vi "LDA_cold_wire_Corr_with_ Displacement.vi"() -> (5 "Plug in titles":string[](array[string]), 7 "Plug in values":string[](array[string]))   [LabVIEW 2021]
uses:
  Controls/Inst_type.ctl
  Globals/Meas_global.vi
  <vilib>/Analysis/NI_AALBase.lvlib
panel:
  out "Cold Wire/FFID Index":i32[](array[numeric])
  out "Maximum Delay Time (s)":dbl=0.02 format="%.3f"
  out "X Displacement (mm) Used":dbl
  in  "Default X Displacement (mm)":dbl=4.0
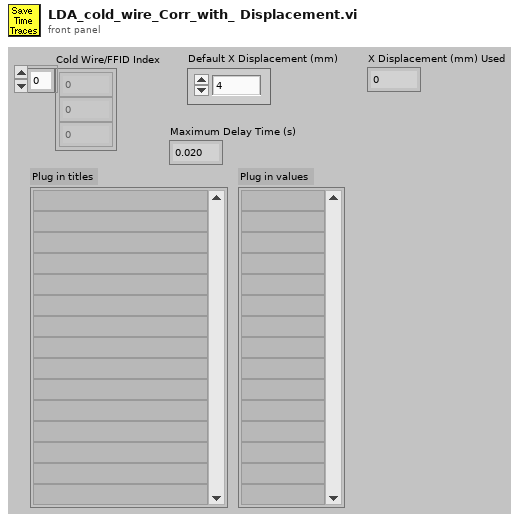
[diagram p1: front panel]
types:
  T1 = typedef "Analysis_info_cluster.ctl" = cluster{"Colour":u32, "Inst type":T2, "Inst name":string, "Symbol":string, "Code name":string, "Extra Info":string, "Inst Array":T3, "Extra Titles":string[], "Extra Values":string[], "U":dbl, "u^2":dbl, "u^3":dbl, "u^4":dbl, "Skew_u":dbl, "Kurt_u":dbl, "Sd Error in Mean":dbl, "% u'/U":dbl, "X":dbl, "Y":dbl, "Z":dbl, "Timescale integral Estimate":dbl, "Sd Error in Variance":dbl, "Calib File":path, "Calib Constants":dbl[], "Output Position":bool, "Stats":enum16{"None", "Basic", "Full"}, "Av Sampling Rate":dbl, "Av No of Samples":dbl, "Total Meas Time (s)":dbl, "ADAM Ch Name":string, "Max value":dbl, "Min value":dbl, "Req Sample Rate Hz":dbl, "Sync Delay Time (s)":dbl, "Ch No":i16, "Device":string, "Use Latest Calib":bool, "Port":string, "Metadata Ch Names":string[], "Metadata Ch Values":string[], "Label":string}
  T2 = typedef "Inst_type.ctl" = enum16{"Raw voltage", "Raw with zero offsetting", "Propeller anemometer", "Pressure Transducer", "Pitot-static tube", "Hot wire", "Cross wire 1", "Cross wire 2", "Generic Linear", "Generic Polynomial", "Generic BackPoly", "Fast FID", "Thermocouple", "Cold wire", "Pulsed Wire", "LDA Vel", "LDA Tran time", "LDA Arr time", "Microphone"}
  T3 = typedef "Instrument_Array.ctl" = enum16{"PWA", "LDA", "Analogue"}
  T4 = typedef "Time_Trace_Cluster.ctl" = cluster{"Weighting":dbl[], "Voltage":dbl[], "Eng Values":dbl[]}
  T5 = typedef "Cross_Moments_Shift_Cluster.ctl" = cluster{"Stats":dbl[], "Resampled No of Samples":i32, "Resampled delta T":dbl, "Cross Correlation":dbl[]}
  T6 = typedef "Shift_Cluster.ctl" = cluster{"Stats":dbl[], "Spectra_Auto":dbl[], "Histogram":dbl[], "Hist Max":dbl, "Hist Min":dbl, "No of Samples":i32, "No in plume":i32, "Weight sum":dbl, "No Of Hist bins":i32, "TimeTrace Max":dbl, "Time Trace Min":dbl, "Trace St Deviation":dbl}
  T7 = typedef "Correlation_cluster1.ctl" = cluster{"U inst":string, "uw":dbl, "u^2w":dbl, "uw^2":dbl, "uw/u'w'":dbl, "W inst":string, "uw^3":dbl, "u^3w":dbl, "u^2w^2":dbl, "Index U":i32, "Index W":i32, "Error info":string[], "Paired Sampling Rate (Hz)":dbl, "u^2 Paired":dbl, "w^2 Paired":dbl, "Time Window (ms)":dbl}
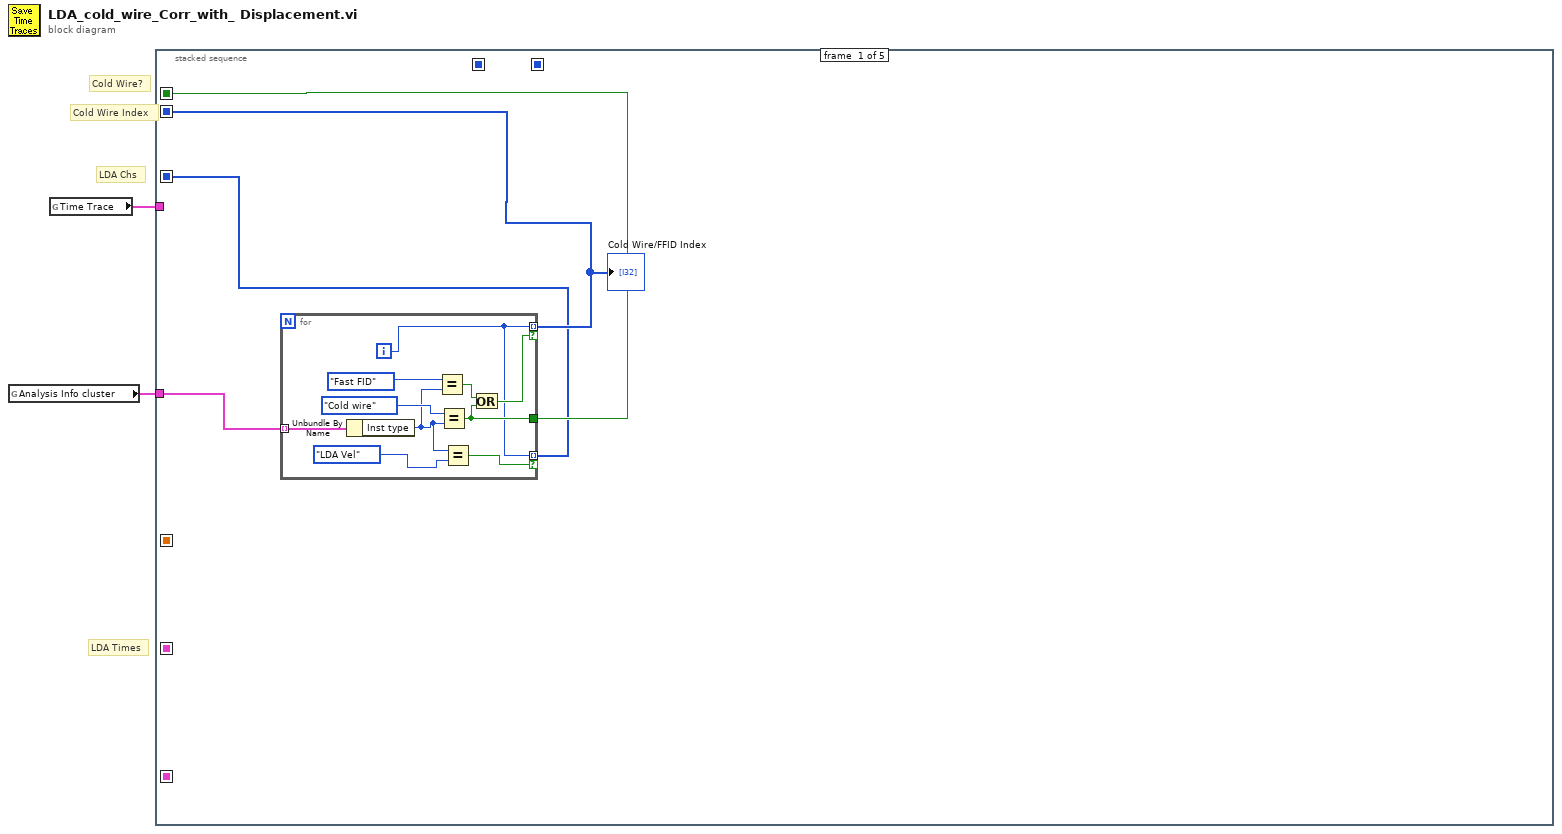
[diagram p0: block diagram]
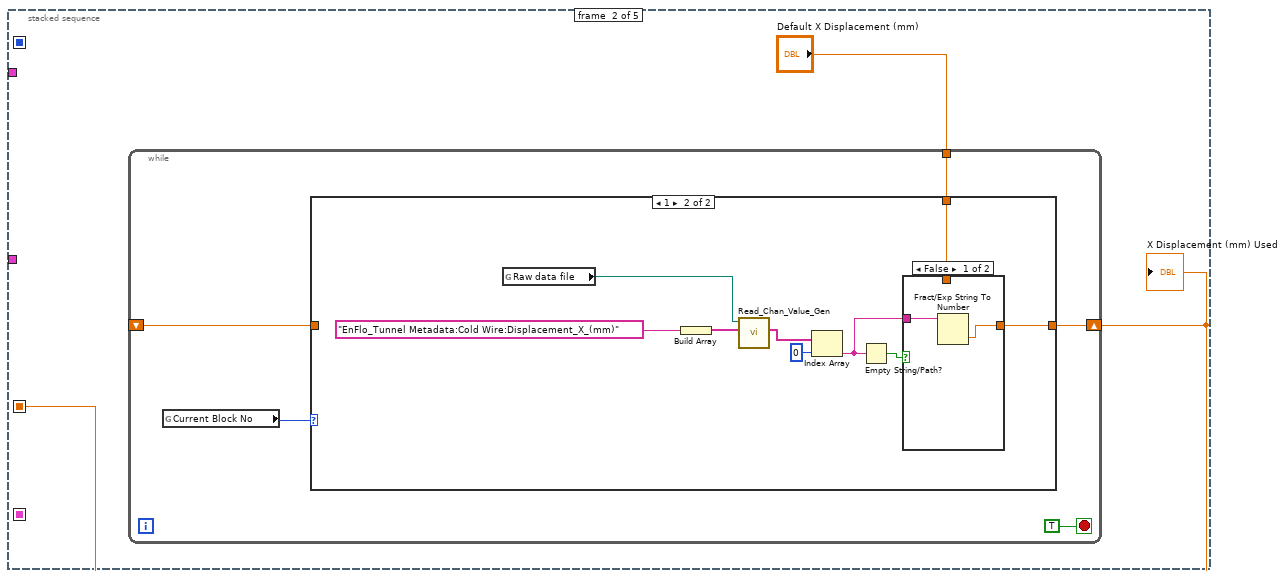
[diagram p2: hidden frame]
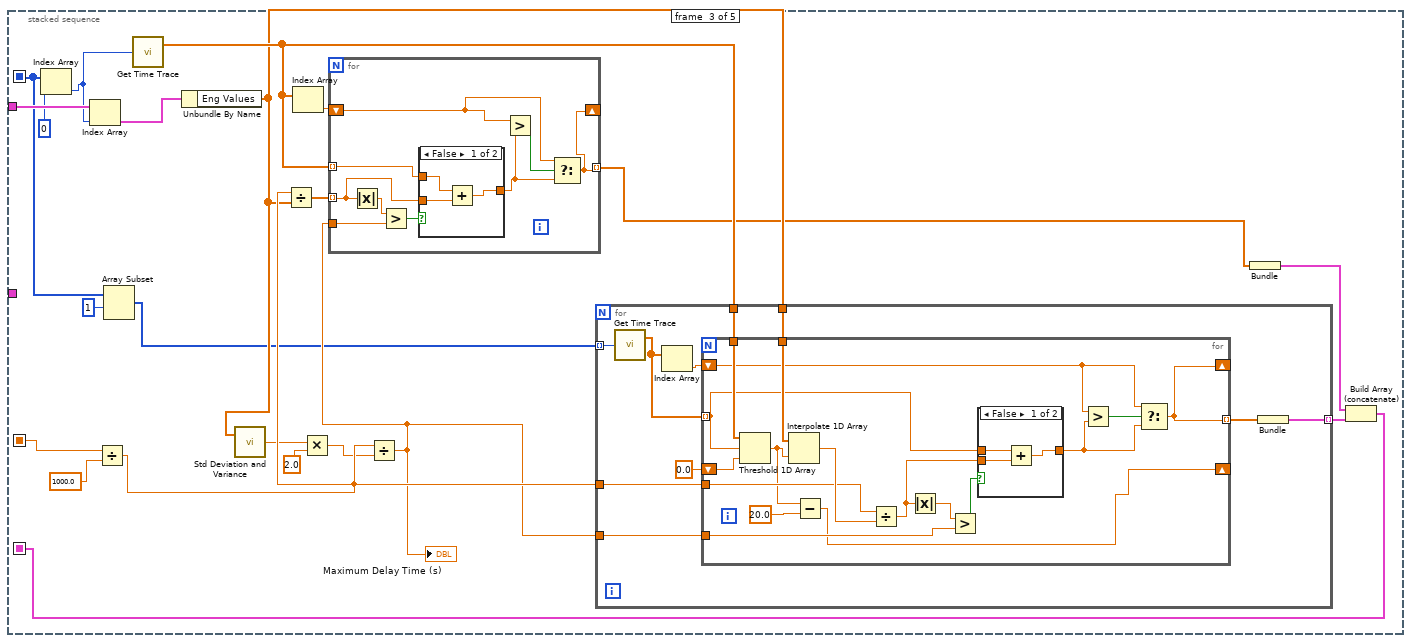
[diagram p5: hidden frame]
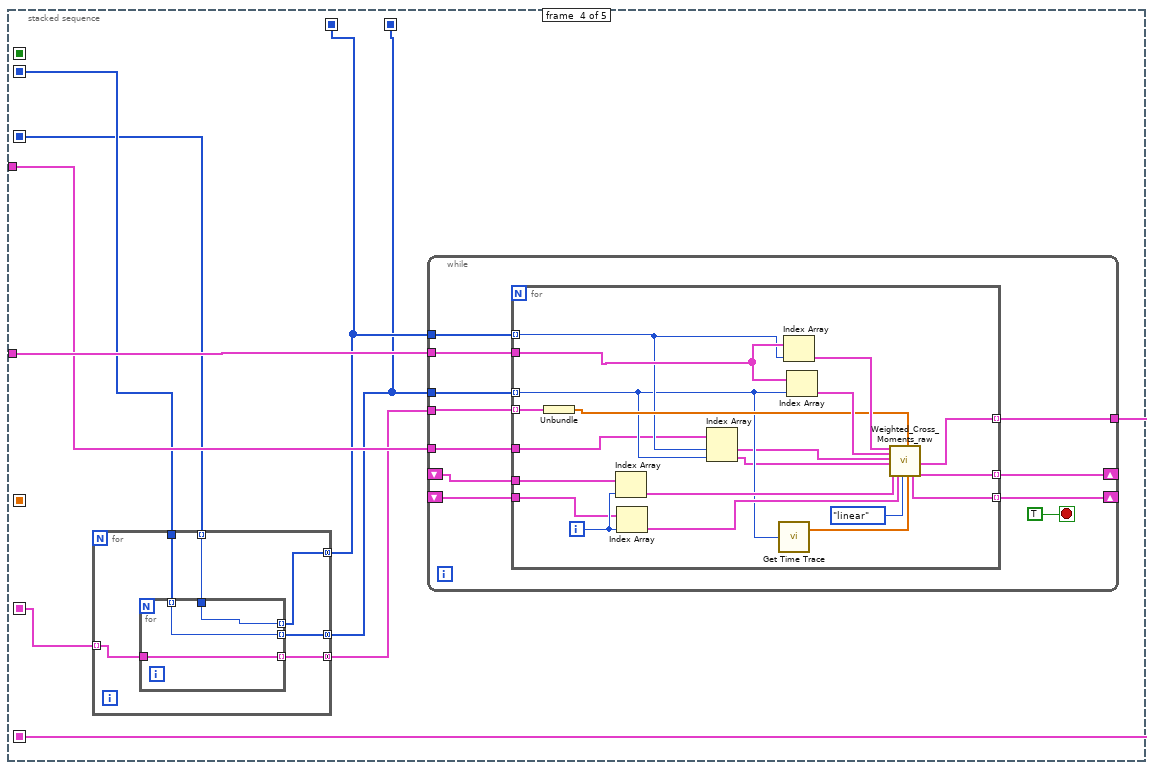
[diagram p8: hidden frame]
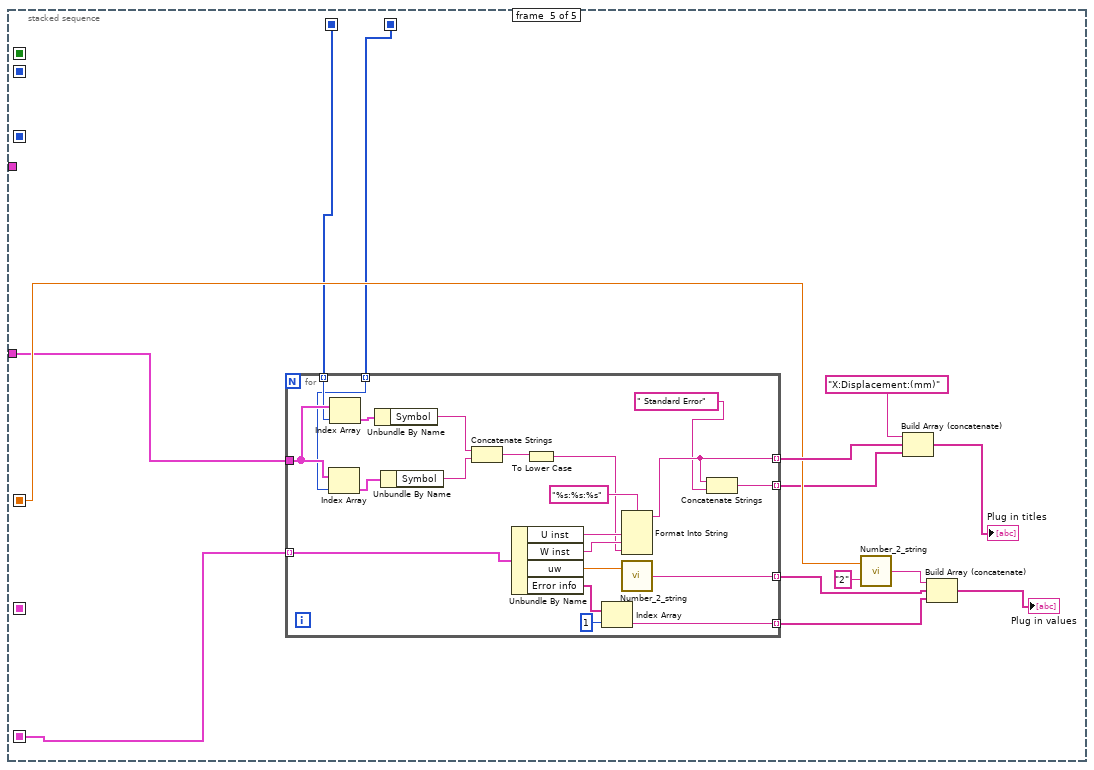
[diagram p9: hidden frame]
diagram:
  # "LDA Chs"
  # "Cold Wire Index"
  # "Cold Wire?"
  # "LDA Times"
  n1 = global read "Meas_global.vi" "Analysis Info cluster"() -> (w1:T1[])
  n2 = global read "Meas_global.vi" "Time Trace"() -> (w2:T4[])
  n3 = stacked-sequence {
    seq-local: [_ _ _ w111 _] -> [_ _ _ _ w155]
    seq-local: [_ _ w37 _ _] -> [_ _ _ w108 _]
    seq-local: [_ w17 _ _ _] -> [_ _ w55 _ w158]
    seq-local: [w5 _ _ _ _] -> [_ _ _ w107 _]
    seq-local: [w4 _ _ _ _] -> [_ _ _ _ _]
    seq-local: [w3 _ _ _ _] -> [_ _ w43 w105 _]
    seq-local: [_ _ _ w104 _] -> [_ _ _ _ w153]
    seq-local: [_ _ _ w103 _] -> [_ _ _ _ w152]
    tunnel: w2 -> [_ _ w46 w109 _]
    tunnel: w1 -> [w6 _ _ w110 w154]
    frame #0 {
      n4 = for {
        tunnel: w6 -> [w16] mode=indexing
        tunnel: [w8] -> w5 mode=indexing if=w11
        tunnel: [w12] -> w4
        tunnel: [w8] -> w3 mode=indexing if=w7
        i -> [w8]
        n5 = Unbundle By Name(w16) -> ("Inst type"=w10:T2)
        n6 = Equal?(x=Inst_type."Fast FID" ("Inst type"), y=w10) -> (x = y?=w13:bool)
        n7 = Equal?(x=Inst_type."Cold wire" ("Inst type"), y=w10) -> (x = y?=w12:bool)
        n8 = Equal?(x=w10, y=Inst_type."LDA Vel" ("Inst type")) -> (x = y?=w7:bool)
        n9 = Or(x=w13, y=w12) -> (x .or. y?=w11:bool)
      }
      "Cold Wire/FFID Index" <- w5
    }
    frame #1 {
      n10 = while {
        tunnel: "Default X Displacement (mm)" -> [w22]
        shift-right: [w21] -> w17
        shift-left: _ -> [w20]
        stop <- TRUE stop-if-true
        n11 = global read "Meas_global.vi" "Current Block No"() -> (w23:i32)
        n12 = case shown="1" w23 {
          tunnel: [w24 w27] -> w21
          tunnel: w22 -> [_ w26]
          tunnel: w20 -> [w24 _]
          frame Default {
          }
          frame 1 {
            n13 = global read "Meas_global.vi" "Raw data file"() -> (w31:path)
            n14 = Build Array("EnFlo_Tunnel Metadata:Cold Wire:Displacement_X_(mm)") -> (w32:string[])
            n15 = call "Read_Chan_Value_Gen.vi"("Desired Ch Names"=w32, "Raw data file"=w31) -> ("Values"=w30:string[])  [unwired: 9 in]
            n16 = Index Array(array=w30, index=0) -> (element=w25:string)
            n17 = Empty String/Path?(string/path=w25) -> (empty?=w28:bool)
            n18 = case shown="False" w28 {
              tunnel: [w34 w36] -> w27
              tunnel: w26 -> [_ w36]
              tunnel: w25 -> [w35 _]
              frame False {
                n19 = Fract/Exp String To Number(string=w35) -> (number=w34:dbl)  [unwired: 3 in, 1 out]
              }
              frame True {
              }
            }
          }
        }
      }
      "X Displacement (mm) Used" <- w17
    }
    frame #2 {
      n20 = Index Array(array=w43, index=0) -> (element=w44:i32)
      n21 = Index Array(array=w46, index=w44) -> (element=w57:T4)
      n22 = Divide(x=w55, y=1000.0) -> (x/y=w56:dbl)
      n23 = Array Subset(array=w43, index=1) -> (w41:i32[])  [unwired: 1 in]
      n24 = call "Get Time Trace.vi"("Channel Index"=w44) -> ("Time (s)"=w54:dbl[])  [unwired: 1 out]
      n25 = Unbundle By Name(w57) -> ("Eng Values"=w51:dbl[])
      n26 = call <vilib>:"Std Deviation and Variance.vi"("X"=w51) -> ("standard deviation"=w50:dbl)  [unwired: 1 in, 2 out]
      n27 = Divide(x=w56, y=w51) -> (x/y=w53:dbl[])
      n28 = Index Array(array=w54) -> (element=w52:dbl)  [unwired: 1 in]
      n29 = Multiply(x=w50, y=2.0) -> (x*y=w48:dbl)
      n30 = Divide(x=w56, y=w48) -> (x/y=w47:dbl)
      "Maximum Delay Time (s)" <- w47
      n31 = for {
        tunnel: w53 -> [w90] mode=indexing
        tunnel: [w94] -> w40 mode=indexing
        tunnel: w54 -> [w91] mode=indexing
        tunnel: w47 -> [w97]
        shift-right: [w94] -> _
        shift-left: w52 -> [w95]
        n32 = Absolute Value(x=w90) -> (abs(x)=w98:dbl)
        n33 = Greater?(x=w98, y=w97) -> (0:w93:bool)
        n34 = case shown="False" w93 {
          tunnel: w91 -> [w101 w102]
          tunnel: [w100 w102] -> w92
          tunnel: w90 -> [w99 _]
          frame False {
            n35 = Add(x=w101, y=w99) -> (x+y=w100:dbl)
          }
          frame True {
          }
        }
        n36 = Greater?(x=w95, y=w92) -> (0:w96:bool)
        n37 = Select(t=w95, s=w96, f=w92) -> (s? t:f=w94:dbl)
      }
      n38 = for {
        tunnel: w56 -> [w68]
        tunnel: w54 -> [w67]
        tunnel: [w59] -> w39 mode=indexing
        tunnel: w51 -> [w64]
        tunnel: w47 -> [w63]
        tunnel: w41 -> [w61] mode=indexing
        n39 = call "Get Time Trace.vi"("Channel Index"=w61) -> ("Time (s)"=w66:dbl[])  [unwired: 1 out]
        n40 = Index Array(array=w66) -> (element=w65:dbl)  [unwired: 1 in]
        n41 = for {
          tunnel: w67 -> [w85]
          tunnel: w66 -> [w81] mode=indexing
          tunnel: w64 -> [w84]
          tunnel: w68 -> [w82]
          tunnel: [w76] -> w60 mode=indexing
          tunnel: w63 -> [w79]
          shift-right: [w76] -> _
          shift-left: w65 -> [w77]
          shift-right: [w69] -> _
          shift-left: 0.0 -> [w72]
          n42 = Threshold 1D Array(1:w72, 2:w81, 3:w85) -> (0:w71:dbl)
          n43 = Interpolate 1D Array(1:w71, 2:w84) -> (0:w83:dbl)
          n44 = Subtract(x=w71, y=20.0) -> (x-y=w69:dbl)
          n45 = Divide(x=w82, y=w83) -> (x/y=w74:dbl)
          n46 = Absolute Value(x=w74) -> (abs(x)=w80:dbl)
          n47 = Greater?(x=w80, y=w79) -> (0:w73:bool)
          n48 = case shown="False" w73 {
            tunnel: w81 -> [w88 w89]
            tunnel: [w87 w89] -> w75
            tunnel: w74 -> [w86 _]
            frame False {
              n49 = Add(x=w88, y=w86) -> (x+y=w87:dbl)
            }
            frame True {
            }
          }
          n50 = Greater?(x=w77, y=w75) -> (0:w78:bool)
          n51 = Select(t=w77, s=w78, f=w75) -> (s? t:f=w76:dbl)
        }
        n52 = Bundle(w60) -> (w59:cluster{dbl[]})  [unwired: 1 in]
      }
      n53 = Bundle(w40) -> (w38:cluster{dbl[]})  [unwired: 1 in]
      n54 = Build Array (concatenate)(w38, w39) -> (w37:cluster{dbl[]}[])
    }
    frame #3 {
      n55 = for {
        tunnel: w108 -> [w114] mode=indexing
        tunnel: w107 -> [w117]
        tunnel: [w116] -> w103 mode=concatenating
        tunnel: [w115] -> w106 mode=concatenating
        tunnel: w105 -> [w113] mode=indexing
        tunnel: [w112] -> w104 mode=concatenating
        n56 = for {
          tunnel: w117 -> [w120] mode=indexing
          tunnel: [w120] -> w116 mode=indexing
          tunnel: [w119] -> w115 mode=indexing
          tunnel: w114 -> [w119]
          tunnel: w113 -> [w118]
          tunnel: [w118] -> w112 mode=indexing
        }
      }
      n57 = while {
        shift-right: [w131] -> _
        shift-left: _ -> [w123]
        tunnel: [w129] -> w111
        tunnel: w110 -> [w128]
        shift-right: [w126] -> _
        shift-left: _ -> [w127]
        tunnel: w103 -> [w125]
        tunnel: w109 -> [w124]
        tunnel: w106 -> [w122]
        tunnel: w104 -> [w121]
        stop <- TRUE stop-if-true
        n58 = for {
          tunnel: [w151] -> w131 mode=indexing
          tunnel: [w148] -> w129 mode=indexing
          tunnel: w128 -> [w147]
          tunnel: w127 -> [w143]
          tunnel: [w146] -> w126 mode=indexing
          tunnel: w125 -> [w135] mode=indexing
          tunnel: w121 -> [w136] mode=indexing
          tunnel: w124 -> [w134]
          tunnel: w123 -> [w144]
          tunnel: w122 -> [w138] mode=indexing
          i -> [w145]
          n59 = Unbundle(w138) -> (w137:dbl[])
          n60 = Index Array(array=w144, index=w145) -> (element=w142:T5)
          n61 = Index Array(array=w143, index=w145) -> (element=w141:T6)
          n62 = Index Array(array=w134, index #1=w136, index #2=w135) -> (element #1=w133:T4, element #2=w132:T4)
          n63 = call "Get Time Trace.vi"("Channel Index"=w135) -> ("Time (s)"=w140:dbl[])  [unwired: 1 out]
          n64 = Index Array(array=w147, index=w136) -> (element=w150:T1)
          n65 = Index Array(array=w147, index=w135) -> (element=w149:T1)
          n66 = call "Weighted_Cross_Moments_raw.vi"("AI Cluster 1"=w150, "AI Cluster 2"=w149, "Time Cluster 1"=w133, "Time Cluster 2"=w132, "Shift Cluster In"=w142, "Shift Input"=w141, "interp. method"=enum16{"nearest", "linear"}."linear", "Time (s) 1"=w137, "Time (s) 2"=w140) -> ("Shift Output"=w146:T6, "output cluster"=w148:T7, "Shift Cluster Out"=w151:T5)  [unwired: 8 in]
        }
      }
    }
    frame #4 {
      n67 = for {
        tunnel: [w186] -> w162 mode=indexing
        tunnel: w155 -> [w185] mode=indexing
        tunnel: [w178] -> w164 mode=indexing
        tunnel: [w176] -> w157 mode=indexing
        tunnel: [w175] -> w156 mode=indexing
        tunnel: w154 -> [w173]
        tunnel: w153 -> [w167] mode=indexing
        tunnel: w152 -> [w166] mode=indexing
        n68 = Index Array(array=w173, index=w166) -> (element=w174:T1)
        n69 = Index Array(array=w173, index=w167) -> (element=w172:T1)
        n70 = Unbundle By Name(w172) -> ("Symbol"=w171:string)
        n71 = Unbundle By Name(w174) -> ("Symbol"=w170:string)
        n72 = Concatenate Strings(w171, w170) -> (w169:string)
        n73 = Unbundle By Name(w185) -> ("U inst"=w183:string, "W inst"=w182:string, "uw"=w184:dbl, "Error info"=w180:string[])
        n74 = To Lower Case(string=w169) -> (all lower case string=w168:string)
        n75 = Index Array(array=w180, index=1) -> (element=w175:string)
        n76 = Format Into String(format string="%s:%s:%s", w183, w182, w168) -> (resulting string=w178:string)  [unwired: 2 in, 1 out]
        n77 = call "Number_2_string.vi"("number"=w184) -> ("String"=w186:string)  [unwired: 1 in]
        n78 = Concatenate Strings(w178, " Standard Error") -> (w176:string)
      }
      n79 = call "Number_2_string.vi"("precision"="2", "number"=w158) -> ("String"=w161:string)
      n80 = Build Array (concatenate)("X:Displacement:(mm)", w164, w157) -> (→"Plug in titles":string[])
      n81 = Build Array (concatenate)(w161, w162, w156) -> (→"Plug in values":string[])
    }
  }
